vi "libssh2_knownhost_writeline.vi"(7 "buffer length (4096)":u32=4096, 8 "error in (no error)":errorcluster, 9 "type (OpenSSH)":T2, 10 "host key":T1, 11 "host key database":T3) -> (0 "error out":errorcluster, 2 "line":string)   [LabVIEW 2013, in "libssh2.lvlib"]
doc: "Write a host key to a string."
uses:
  libssh2.lvlib
  Host Key Database Refnum.ctl
  Host Key File Type.ctl
  Host Key Refnum.ctl
  Not A Host Key Database.vi
  <vilib>/Utility/error.llb/Error Cluster From Error Code.vi
  Not A Host Key.vi
  Global Settings.vi
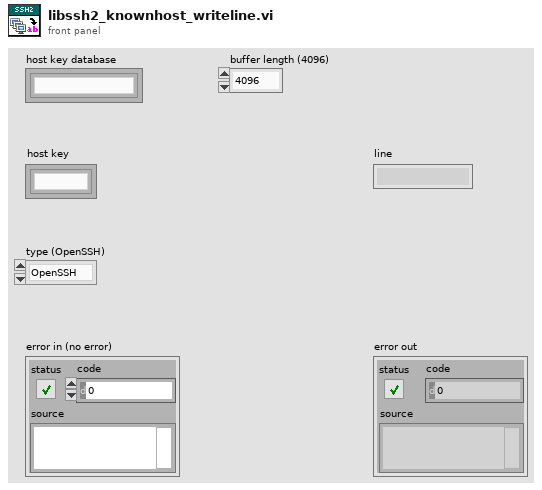
[diagram p1: front panel]
types:
  T1 = typedef "libssh2.lvlib/Host Key Refnum.ctl" = refnum<k1>
  T2 = typedef "libssh2.lvlib/Host Key File Type.ctl" = enum16{"OpenSSH"}
  T3 = typedef "libssh2.lvlib/Host Key Database Refnum.ctl" = refnum<k1>
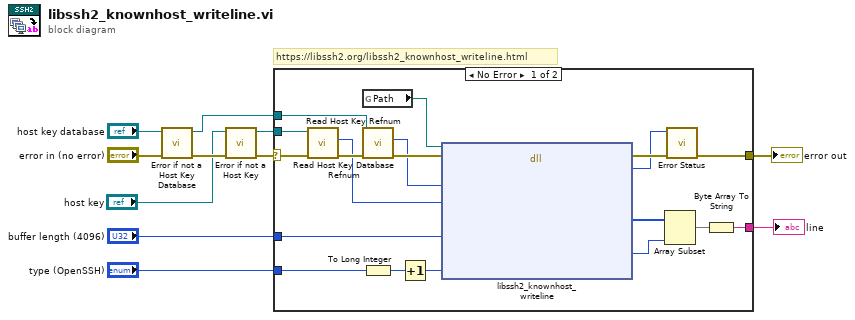
[diagram p0: block diagram]
diagram:
  # "https://libssh2.org/libssh2_knownhost_writeline.html"
  n1 = call "Error if not a Host Key Database.vi"("error in (no error)"="error in (no error)", "host key database"="host key database") -> ("error out"=w8:errorcluster, "host key database out"=w6:T3)  [unwired: 8 in]
  n2 = call "Error if not a Host Key.vi"("error in (no error)"=w8, "host key"="host key") -> ("error out"=w3:errorcluster, "host key out"=w1:T1)  [unwired: 8 in]
  n3 = case shown="No Error" w3 {
    selector: w3 -> [w29 w31]
    tunnel: [w28 w31] -> w11
    tunnel: "type (OpenSSH)" -> [w30 _]
    tunnel: w6 -> [w27 _]
    tunnel: "buffer length (4096)" -> [w19 _]
    tunnel: [w15 _] -> w4
    tunnel: w1 -> [w12 _]
    frame No Error {
      n4 = call "Read Host Key Refnum.vi"("error in (no error)"=w29, "host key"=w12) -> ("error out"=w14:errorcluster, "libssh2_knownhost*"=w13:u64)  [unwired: 8 in]
      n5 = global read "Global Settings.vi" "Path"() -> (w23:path)
      n6 = call "Read Host Key Database Refnum.vi"("error in (no error)"=w14, "host key database"=w27) -> ("error out"=w25:errorcluster, "LIBSSH2_KNOWNHOSTS*"=w24:u64)  [unwired: 8 in]
      n7 = To Long Integer(number=w30) -> (32bit integer=w21:i32)
      n8 = Increment(x=w21) -> (x+1=w20:i32)
      n9 = dll-call lib="?" fn="libssh2_knownhost_writeline"(path in=w23, error in=w25, "hosts"=w24, "known"=w13, "buflen"=w19, "type"=w20) -> (error out=w26:errorcluster, "return value"=w22:i32, "buffer"=w18:u8[], "outlen"=w17:i32)  [unwired: 7 in, 1 out]
      n10 = Array Subset(array=w18, length=w17) -> (w16:u8[])  [unwired: 1 in]
      n11 = call "Error Status.vi"("error in (no error)"=w26, "return value"=w22) -> ("error out"=w28:errorcluster)  [unwired: 8 in, 1 out]
      n12 = Byte Array To String(unsigned byte array=w16) -> (string=w15:string)
    }
    frame Error {
    }
  }
  "error out" <- w11
  "line" <- w4
